vi "Obtain tagDB DVR.vi"(8 "error in (no error)":errorcluster, 10 "name":string) -> (0 "error out":errorcluster, 3 "TagDB":refnum<k1>)   [LabVIEW 2017, in "TagDB.lvlib"]
uses:
  TagDB.lvlib
  Typedef/tagdb-data.ctl
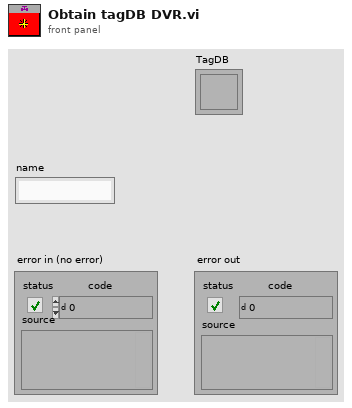
[diagram p1: front panel]
types:
  T1 = typedef "TagDB.lvlib/tagdb-data.ctl" = cluster{"tag-map":variant, "timestamp-map":variant, "namecacher-map":variant, "DataTypeCacher-map":variant, "Tag Adding Lock?":bool, "Global Change Timestamp":timestamp, "Item Change Timestamp":timestamp, "name":string, "Global Change Flag":u64, "Item Change Flag":u64}
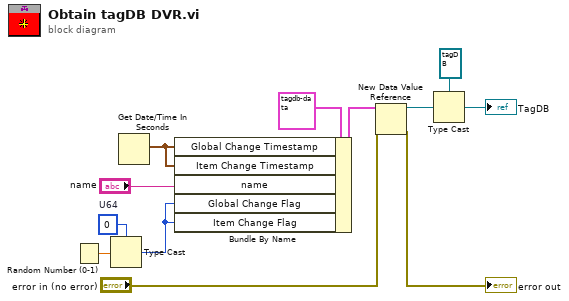
[diagram p0: block diagram]
diagram:
  w2 = u64 0  # U64
  n1 = Random Number (0-1)() -> (number: 0 to 1=w3:dbl)
  n2 = Type Cast(type=w2, x=w3) -> (*(type *) &x=w1:u64)
  n3 = Get Date/Time In Seconds() -> (seconds since 1Jan1904=w5:timestamp)
  n4 = Bundle By Name(cluster=T1 {"tag-map"=variant, "timestamp-map"=variant, "namecacher-map"=variant, "DataTypeCacher-map"=variant, "Tag Adding Lock?"=FALSE, "Global Change Timestamp"=timestamp(0 s since 1904-01-01), "Item Change Timestamp"=timestamp(0 s since 1904-01-01), "name"="", "Global Change Flag"=0, "Item Change Flag"=0}, "Global Change Timestamp"=w5, "Item Change Timestamp"=w5, "name"="name", "Global Change Flag"=w1, "Item Change Flag"=w1) -> (w6:T1)
  n5 = New Data Value Reference(data value=w6, error in="error in (no error)") -> (data value reference=w10:refnum<data-value>, error out=→"error out":errorcluster)
  n6 = Type Cast(type=refnum<k1> refnum ("TagDB"), x=w10) -> (*(type *) &x=→"TagDB":refnum<k1>)
